vi "Water Tank 2.vi"() -> ()   [LabVIEW 2024]
panel:
  in  "stop":bool
  out "Boolean":bool
  out "Tank":dbl(slide) scale=0.0..100.0
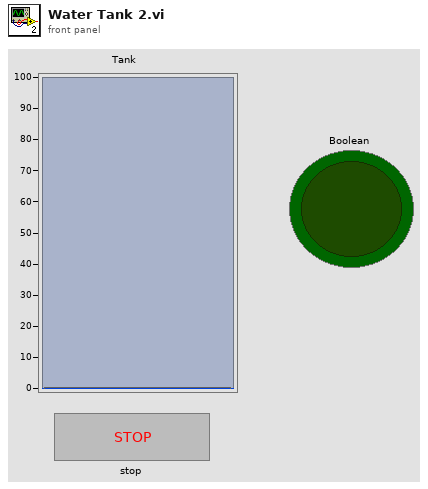
[diagram p1: front panel]
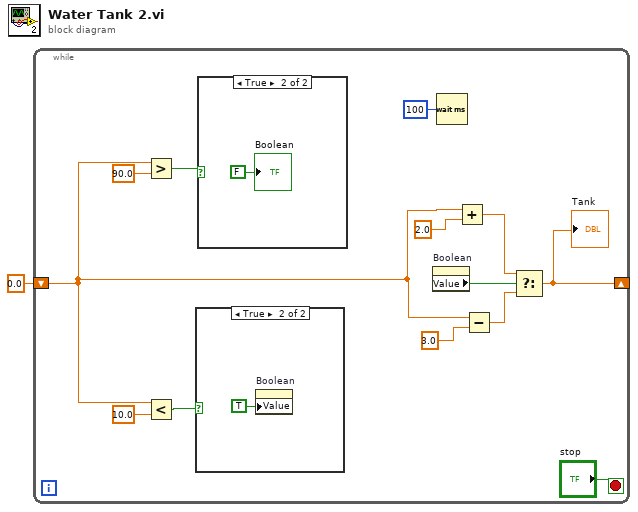
[diagram p0: block diagram]
diagram:
  n1 = while {
    shift-right: [w3] -> _
    shift-left: 0.0 -> [w6]
    stop <- "stop" stop-if-true
    n2 = Greater?(x=w6, y=90.0) -> (0:w5:bool)
    n3 = Less?(x=w6, y=10.0) -> (x < y?=w2:bool)
    n4 = case shown="True" w2 {
      frame False {
      }
      frame True {
        n5 = property on="Boolean" class="Bool (strict)"("Value"=TRUE ("Boolean")) -> ()  [unwired: 2 in, 2 out]
      }
    }
    n6 = case shown="True" w5 {
      frame False {
      }
      frame True {
        "Boolean" <- FALSE ("Boolean")
      }
    }
    n7 = property on="Boolean" class="Bool (strict)"() -> ("Value"=w11:bool)  [unwired: 2 in, 2 out]
    n8 = Wait (ms)(milliseconds to wait=u32 100) -> ()  [unwired: 1 out]
    n9 = Add(x=w6, y=2.0) -> (x+y=w9:dbl)
    n10 = Subtract(x=w6, y=3.0) -> (x-y=w7:dbl)
    n11 = Select(t=w9, s=w11, f=w7) -> (s? t:f=w3:dbl)
    "Tank" <- w3
  }
